vi "WS2812 Write N LED.vi"() -> ()   [LabVIEW 2017]
uses:
  IMAQCV/PIIO/Core/PIIO DIO.ctl
  IMAQCV/PIIO.lvlib
panel:
  in  "PIN":T1 items=["L1", "L2"]
  in  "stop":bool
  in  "LED Colors":u32[](array[colorbox])=[16711680, 6618880, 16860]
  in  "LED Start Index":u16
  in  "Number of LEDs":u16=40
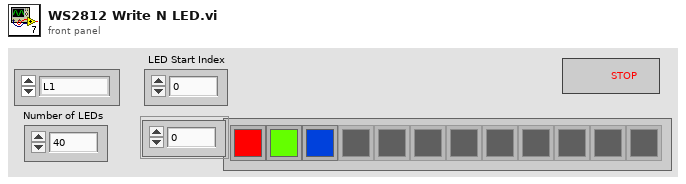
[diagram p1: front panel]
types:
  T1 = typedef "PIIO.lvlib/PIIO DIO.ctl" = u8
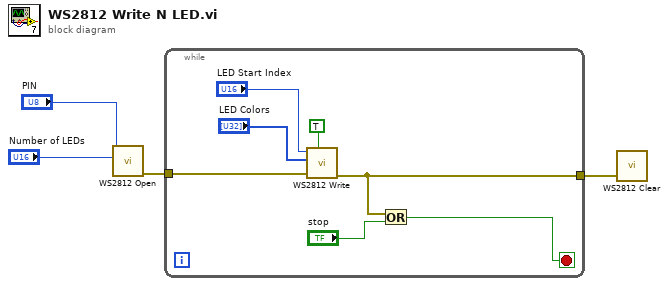
[diagram p0: block diagram]
diagram:
  n1 = call "WS2812 Open.vi"("Number of LEDs"="Number of LEDs", "PIN"="PIN") -> ("Error Out"=w4:errorcluster)  [unwired: 9 in]
  n2 = while {
    tunnel: w4 -> [w11]
    tunnel: [w6] -> w3
    stop <- w8 stop-if-true
    n3 = call "WS2812 Write.vi"("Refresh?"=TRUE, "Error In"=w11, "Colors"="LED Colors", "Start Pixel Index"="LED Start Index") -> ("Error Out"=w6:errorcluster)  [unwired: 7 in]
    n4 = Or(x=w6, y="stop") -> (x .or. y?=w8:bool)
  }
  n5 = call "WS2812 Clear.vi"("Error In"=w3) -> ()  [unwired: 10 in, 1 out]
